vi "MP_LaunchMatlabScript.vi"(8 "error in (no error)":errorcluster, 10 "matlab script name with extension":string) -> (0 "error out":errorcluster, 2 "standard error":string, 3 "standard output":string, 4 "OS Name":string, 5 "computed command line":string)   [LabVIEW 2013]
doc: "Launch matlab with the script passed as parameter. \nThe script and the VI MUST be in the same directory!\n\nThis vi is specially taillored fot the algo 2013 class. Works on OSX, Windows and Linux On Linux, assume Ubuntu (salles CO) and current 2013 \"matlab\" CMD. \nOn OSX, search for the latest release of matlab, see diagram.\nOn Windows, assume \"matlab\" command exists.\n\nThere is demo script if needed, see the diagram to activate it.\n\nChS. 14.5.2013"
uses:
  <vilib>/Utility/sysdir.llb/System Directory Type.ctl
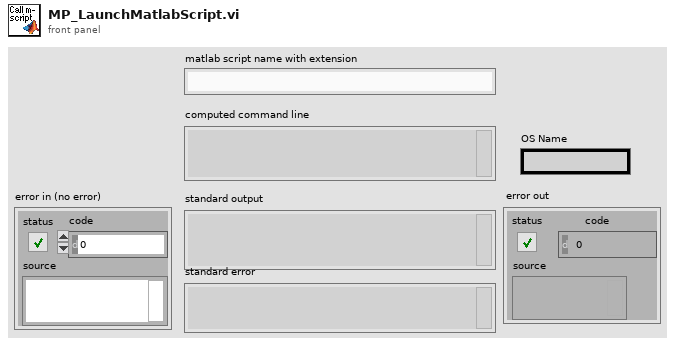
[diagram p1: front panel]
types:
  T1 = enum16{"open", "replace", "create", "open or create", "replace or create", "replace or create with confirmation"}
  T2 = typedef "System Directory Type.ctl" = i32
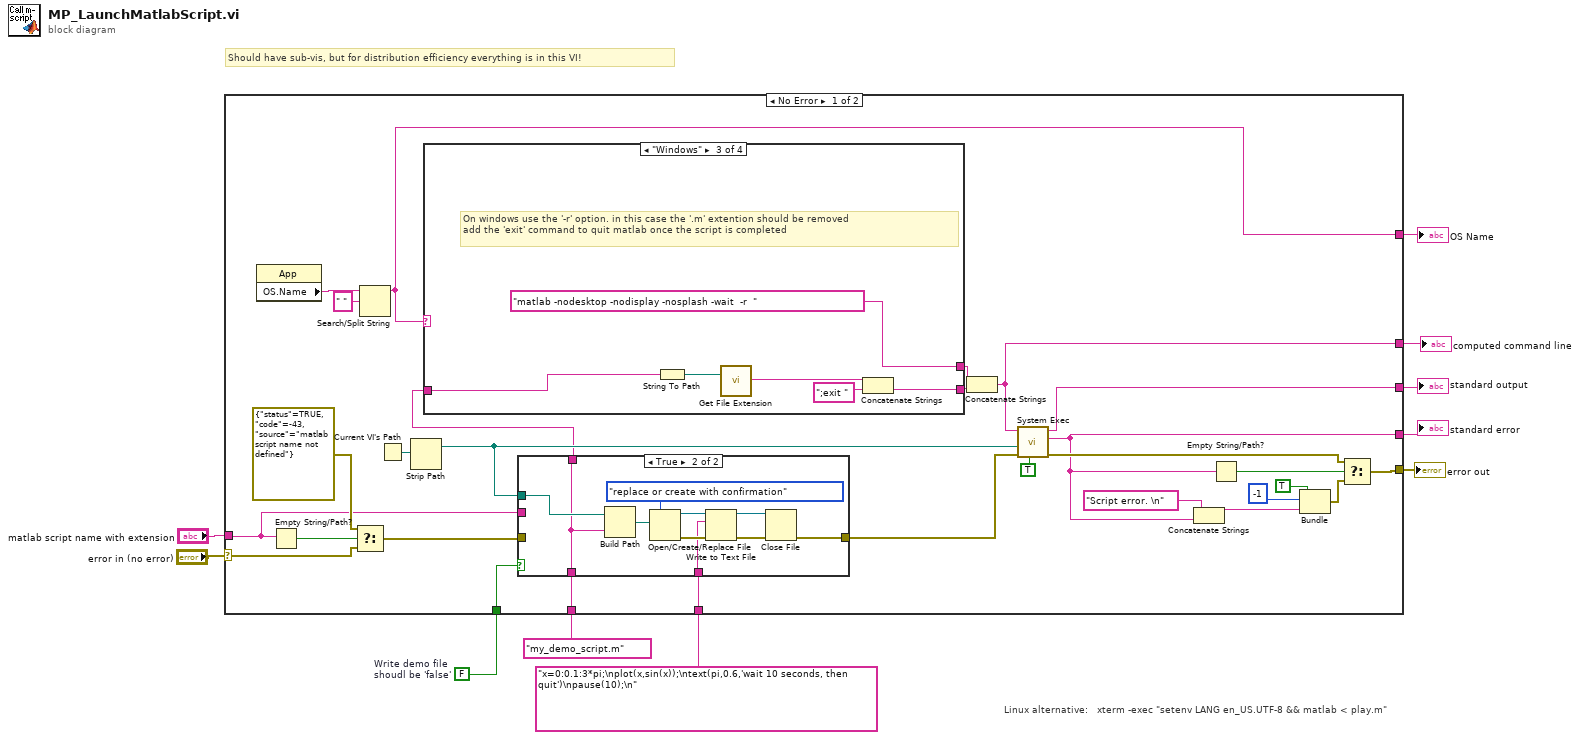
[diagram p0: block diagram]
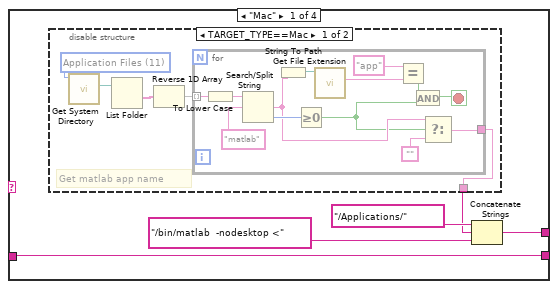
[diagram p3: hidden frame]
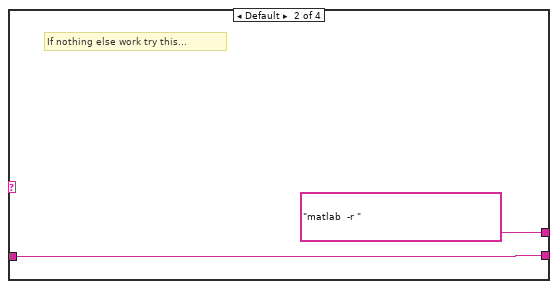
[diagram p5: hidden frame]
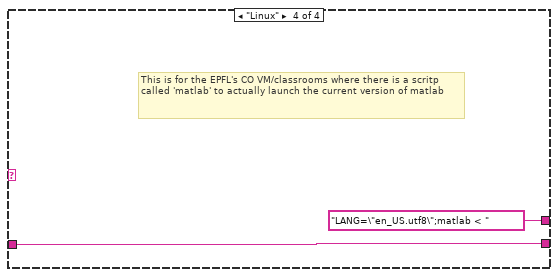
[diagram p6: hidden frame]
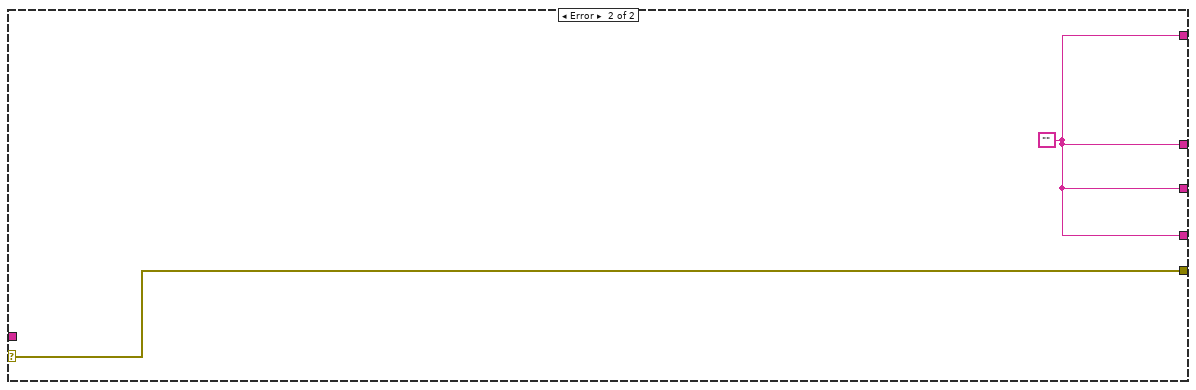
[diagram p7: hidden frame]
diagram:
  w1 = FALSE  # Write demo file shoudl be 'false'
  # "Should have sub-vis, but for distribution efficiency everything is in this VI!"
  # "Linux alternative:   xterm -exec \"setenv LANG en_US.UTF-8 && matlab < play.m\""
  n1 = case shown="No Error" "error in (no error)" {
    selector: "error in (no error)" -> [w34 w86]
    tunnel: [w38 w85] -> w10
    tunnel: [w24 w85] -> w9
    tunnel: [w26 w86] -> w8
    tunnel: "matlab script name with extension" -> [w31 _]
    tunnel: [w29 w85] -> w5
    tunnel: [w16 w85] -> w4
    tunnel: "x=0:0.1:3*pi;\nplot(x,sin(x));\ntext(pi,0.6,'wait 10 seconds, then quit')\npause(10);\n" ("text") -> [w14 _]
    tunnel: "my_demo_script.m" ("name or relative path") -> [w13 _]
    tunnel: w1 -> [w12 _]
    frame No Error {
      n2 = property class="App"() -> ("OS.Name"=w17:string)  [unwired: 2 in, 2 out]
      n3 = Empty String/Path?(string/path=w31) -> (empty?=w35:bool)
      n4 = Select(t=errorcluster {"status"=TRUE, "code"=-43, "source"="matlab script name not defined"} ("error constant"), s=w35, f=w34) -> (s? t:f=w32:errorcluster)
      n5 = Search/Split String(string=w17, search string/char (-)=" ") -> (substring before match=w16:string)  [unwired: 1 in, 2 out]
      n6 = Current VI's Path() -> (path=w39:path)
      n7 = Strip Path(path=w39) -> (stripped path=w36:path)  [unwired: 1 out]
      n8 = case shown="True" w12 {
        tunnel: [w41 w47] -> w37
        tunnel: w36 -> [_ w45]
        tunnel: w32 -> [w41 _]
        tunnel: w31 -> [w40 _]
        tunnel: [w40 w42] -> w19
        tunnel: w14 -> [_ w43]
        tunnel: w13 -> [_ w42]
        frame False {
        }
        frame True {
          n9 = Build Path(base path=w45, name or relative path=w42) -> (appended path=w44:path)
          n10 = Open/Create/Replace File(file path (use dialog)=w44, operation (0:open)=T1."replace or create with confirmation") -> (refnum out=w48:refnum<file>, error out=w51:errorcluster)  [unwired: 4 in, 1 out]
          n11 = Write to Text File(file (use dialog)=w48, text=w43, error in=w51) -> (refnum out=w49:refnum<file>, error out=w50:errorcluster)  [unwired: 1 in, 1 out]
          n12 = Close File(refnum=w49, error in=w50) -> (error out=w47:errorcluster)  [unwired: 1 out]
        }
      }
      n13 = case shown="\"Windows\"" w16 {
        tunnel: [w53 "matlab  -r " ("name or relative path") "matlab -nodesktop -nodisplay -nosplash -wait  -r  " ("name or relative path") "LANG=\"en_US.utf8\";matlab < "] -> w30
        tunnel: w19 -> [w56 w75 w81 w83]
        tunnel: [w56 w75 w78 w83] -> w18
        frame "Mac" {
          n14 = disable-structure shown="TARGET_TYPE==Mac" {
            disable-tunnel: [w57 _] -> w52
            frame condition #0 {
              w61 = T2 11 items=["User Home"=0, "User Desktop"=1, "User Documents"=2, "User Application Data"=3, "User Preferences"=4, "User Temporary"=5, "Public Documents"=6, "Public Application Data"=7, "Public Preferences"=8, "Public Cache"=13, "System Core Libraries"=9, "System Installed Libraries"=10, "Application Files"=11, "Boot Volume Root"=12] ("system directory type")
              # "Get matlab app name"
              n15 = call <vilib>:"Get System Directory.vi"("system directory type"=w61) -> ("system directory"=w58:path)  [unwired: 10 in]
              n16 = List Folder(path=w58) -> (folder names=w60:string[])  [unwired: 3 in, 3 out]
              n17 = Reverse 1D Array(array=w60) -> (reversed array=w59:string[])
              n18 = for {
                tunnel: w59 -> [w74] mode=indexing
                tunnel: [w65] -> w57
                stop <- w67 stop-if-true
                n19 = To Lower Case(string=w74) -> (all lower case string=w73:string)
                n20 = Search/Split String(string=w73, search string/char (-)="matlab") -> (match + rest of string=w64:string, offset of match=w71:i32)  [unwired: 1 in, 1 out]
                n21 = String To Path(string=w64) -> (path=w70:path)
                n22 = Greater Or Equal To 0?(x=w71) -> (x >= 0?=w63:bool)
                n23 = call <vilib>:"Get File Extension.vi"("file"=w70) -> ("lowercase file extension"=w68:string)  [unwired: 7 in, 3 out]
                n24 = Equal?(x="app", y=w68) -> (x = y?=w66:bool)
                n25 = And(x=w66, y=w63) -> (x .and. y?=w67:bool)
                n26 = Select(t=w64, s=w63, f="") -> (s? t:f=w65:string)
              }
            }
            frame condition #1 (active) {
            }
          }
          n27 = Concatenate Strings("/Applications/" ("name or relative path"), w52, "/bin/matlab  -nodesktop <" ("name or relative path")) -> (w53:string)
        }
        frame Default {
          # "If nothing else work try this..."
        }
        frame "Windows" {
          # "On windows use the '-r' option. in this case the '.m' extention should be removed\nadd the 'exit' command to quit matlab once the script is completed"
          n28 = String To Path(string=w81) -> (path=w80:path)
          n29 = call <vilib>:"Get File Extension.vi"("file"=w80) -> ("filename without extension"=w79:string)  [unwired: 7 in, 3 out]
          n30 = Concatenate Strings(w79, ";exit " ("string")) -> (w78:string)
        }
        frame "Linux" {
          # "This is for the EPFL's CO VM/classrooms where there is a scritp called 'matlab' to actually launch the current version of matlab"
        }
      }
      n31 = Concatenate Strings(w30, w18) -> (w29:string)
      n32 = call <vilib>:"System Exec.vi"("run minimized? (F)"=TRUE, "error in (no error)"=w37, "working directory"=w36, "command line"=w29) -> ("error out"=w27:errorcluster, "standard error"=w24:string, "standard output"=w38:string)  [unwired: 4 in, 1 out]
      n33 = Concatenate Strings("Script error. \n" ("source"), w24) -> (w21:string)
      n34 = Empty String/Path?(string/path=w24) -> (empty?=w28:bool)
      n35 = Bundle("status"=TRUE, "code"=-1, w21) -> (w25:cluster{"status":bool, "code":i32, string})  [unwired: 1 in]
      n36 = Select(t=w27, s=w28, f=w25) -> (s? t:f=w26:errorcluster)
    }
    frame Error {
      w85 = "" ("standard error")
    }
  }
  "standard output" <- w10
  "standard error" <- w9
  "error out" <- w8
  "computed command line" <- w5
  "OS Name" <- w4
